vi "Add Section.vi"(7 "GUID (Default Section)":string="03D3BB89-1485-13A6-56005DE6430FF8B7", 8 "error in":errorcluster, 10 "Section Name":string, 11 "Parent Ref in":T1 format="%.0x") -> (0 "error out":errorcluster, 2 "Section Ptr":T1 format="%.0x", 3 "Parent Ref out":T1 format="%.0x")   [LabVIEW 2026, in "NIVS Runtime Configuration File Scripting API.lvlib"]
uses:
  NIVS Runtime Configuration File Scripting API.lvlib
  <vilib>/NI VeriStand/Custom Device API/Custom Device Item Ref.ctl
  <vilib>/NI VeriStand/Custom Device Offline API/Custom Device Offline API.lvlib
  <vilib>/NI VeriStand/Custom Device API/Custom Device API.lvlib
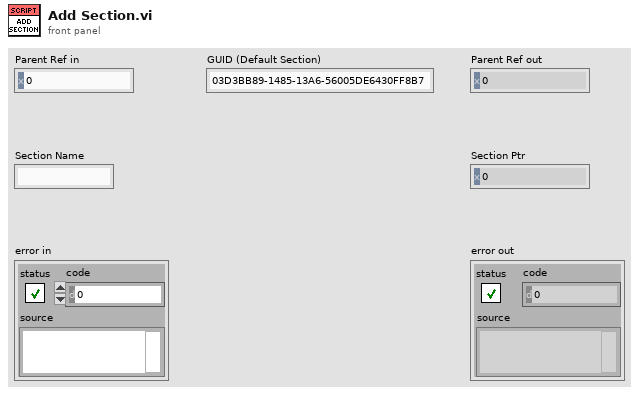
[diagram p1: front panel]
types:
  T1 = typedef "Custom Device API.lvlib/Custom Device Item Ref.ctl" = u64
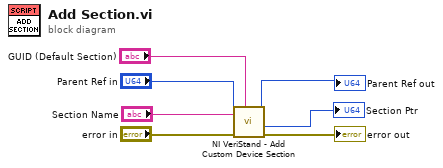
[diagram p0: block diagram]
diagram:
  n1 = call <vilib>:"NI VeriStand - Add Custom Device Section.vi"("GUID (Default Section)"="GUID (Default Section)", "error in (no error)"="error in", "Section Name"="Section Name", "Parent Ref in"="Parent Ref in") -> ("error out"=→"error out":errorcluster, "Section Ptr"=→"Section Ptr":T1, "Parent Ref out"=→"Parent Ref out":T1)  [unwired: 4 in, 1 out]
